vi "FPGA_pwm.vi"() -> ()   [LabVIEW 2018]
uses:
  <vilib>/rvi/Emulation/niFpgaGetClockAttributes.vi
  <vilib>/rvi/Emulation/niFpgaSctlEmulationGetInTimedLoop.vi
  <vilib>/rvi/Emulation/niFpgaEmulationReportErrorSimple.vi
  <vilib>/rvi/eio/common/nirviEmuTemplateMethod_errors.vi
  <vilib>/rvi/Emulation/niFpgaProcessEmulError.vi
  <vilib>/rvi/Emulation/niFpgaCriticalErrorInLSC.vi
  <vilib>/eio/EIONode/EIONode.xnode
panel:
  in  "Count(mSec)":u32
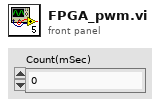
[diagram p1: front panel]
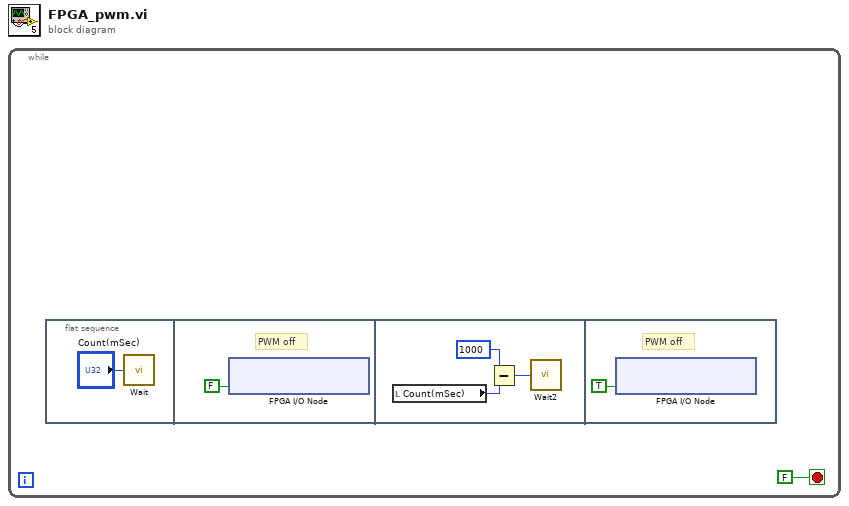
[diagram p0: block diagram]
diagram:
  n1 = while {
    stop <- FALSE stop-if-true
    n2 = flat-sequence {
      frame #0 {
        n3 = call "Wait"("Count(mSec)"="Count(mSec)") -> ()  [unwired: 1 out]
      }
      frame #1 {
        # "PWM off"
        n4 = xnode "FPGA I/O Node"("ConnectorA/DIO8"=FALSE) -> ()  [unwired: 1 in, 1 out]
      }
      frame #2 {
        n5 = local read "Count(mSec)"() -> (w5:u32)
        n6 = Subtract(x=i16 1000, y=w5) -> (x-y=w4:u32)
        n7 = call "Wait2"("Count(mSec)"=w4) -> ()  [unwired: 1 out]
      }
      frame #3 {
        # "PWM off"
        n8 = xnode "FPGA I/O Node"("ConnectorA/DIO8"=TRUE) -> ()  [unwired: 1 in, 1 out]
      }
    }
  }
